vi "TEMOCR-Initialize Stimuli.vi"(0 "Data folder":path, 5 "Params":T2, 7 "AO in":T1, 11 "error in (no error)":errorcluster) -> (8 "AO out":T1, 15 "error out":errorcluster)   [LabVIEW 2015]
uses:
  Typedefs/TEMOCR-Parameters.ctl
  Typedefs/TEMOCR-Probe.ctl
  Typedefs/TEMOCR-Elicitor.ctl
  Human Studies/SFM Frontend/LV Source/Typedefs/HSTS-Transducer.ctl
  Typedefs/TEMOCR-Sequence.ctl
  Typedefs/TEMOCR-Analysis.ctl
  Typedefs/TEMOCR-AO Data.ctl
  Signal Synthesis VIs/3rd Generation/XControls/Stimulus Channel (G3)/Full Stimulus Channel Data.ctl
  Signal Synthesis VIs/3rd Generation/XControls/Waveform XControls/Waveform (G3)/Waveform Data.ctl
  Signal Synthesis VIs/3rd Generation/Waveform VIs/Waveform Enum (V3).ctl
  Signal Synthesis VIs/3rd Generation/XControls/Waveform XControls/Tone (G3)/Tone.Properties.ctl
  Signal Synthesis VIs/Waveform VIs/Pulse Train VIs/Pulse Train Params.ctl
  Signal Synthesis VIs/Waveform VIs/Pulse Train VIs/Pulse Polarity.ctl
  Signal Synthesis VIs/Waveform VIs/Pulse Train VIs/PT-Continuous State.ctl
  Signal Synthesis VIs/3rd Generation/Waveform VIs/Noise VIs/Noise (G3).ctl
  Signal Synthesis VIs/3rd Generation/Waveform VIs/Noise VIs/Noise (G3).Properties.ctl
  Signal Synthesis VIs/3rd Generation/Waveform VIs/Noise VIs/Noise (G3).Data.ctl
  Signal Synthesis VIs/Waveform VIs/File VIs/StimFile-Params.ctl
  Signal Synthesis VIs/Waveform VIs/FM Sweep VIs/FM Sweep Params.ctl
  Signal Synthesis VIs/Waveform VIs/Chirp Train VIs/Chirp Train.ctl
  Signal Synthesis VIs/Waveform VIs/Chirp Train VIs/Chirp Train Params.ctl
  Signal Synthesis VIs/Waveform VIs/Complex Tone VIs/CT-Params.ctl
  Signal Synthesis VIs/Waveform VIs/Complex Tone VIs/CT-Phase Enum.ctl
  Signal Synthesis VIs/Waveform VIs/Complex Tone VIs/CT-Runtime Data.ctl
  Signal Synthesis VIs/3rd Generation/XControls/Waveform XControls/FM Tone/Data.ctl
  Signal Synthesis VIs/3rd Generation/XControls/Waveform XControls/Vowel/Vowel.Properties.ctl
  Signal Synthesis VIs/3rd Generation/Waveform VIs/Ramp VIs/Ramp.Properties.ctl
  Signal Synthesis VIs/3rd Generation/XControls/Filter (G3)/Filter Data.ctl
  Signal Synthesis VIs/3rd Generation/XControls/Filter (G3)/Filter Type.ctl
  Signal Synthesis VIs/Filter VIs/Filter-Bandwidth Units.ctl
  Signal Synthesis VIs/Controls/Burst XCtl/Burst Data.ctl
  Signal Synthesis VIs/3rd Generation/XControls/Level (G3)/Level Data.ctl
  Signal Synthesis VIs/3rd Generation/XControls/Level (G3)/Level Units (G3).ctl
  Signal Synthesis VIs/3rd Generation/XControls/Advanced Options (G3)/Advanced Options (G3).ctl
  Signal Synthesis VIs/Modulation VIs/SAM VIs/SAM Params.ctl
  Signal Synthesis VIs/3rd Generation/Typedefs/Destination.ctl
  PXI DAQ VIs/DAQ Engine VIs/PXI Globals.vi
  Signal Synthesis VIs/Waveform VIs/Noise VIs/Noise-Globals.vi
  Utility VIs/Math VIs/LinSpace (start-stop-step).vi
  Utility VIs/Math VIs/dB to Linear (1D).vi
  Signal Synthesis VIs/3rd Generation/XControls/Waveform XControls/Tone (G3)/Tone (G3).xctl
  Signal Synthesis VIs/3rd Generation/XControls/Waveform XControls/FM Tone/FM Tone.xctl
  Signal Synthesis VIs/3rd Generation/XControls/Waveform XControls/Vowel/Vowel.xctl
  Signal Synthesis VIs/3rd Generation/XControls/Waveform XControls/Waveform (G3)/Waveform (G3).xctl
  Signal Synthesis VIs/3rd Generation/XControls/Filter (G3)/Filter (G3).xctl
  Signal Synthesis VIs/Controls/Burst XCtl/Burst Control.xctl
  Signal Synthesis VIs/3rd Generation/XControls/Level (G3)/Level (G3).xctl
  Signal Synthesis VIs/3rd Generation/XControls/Advanced Options (G3)/Advanced Options (G3).xctl
  Signal Synthesis VIs/3rd Generation/XControls/Stimulus Channel (G3)/Stimulus Channel (G3).xctl
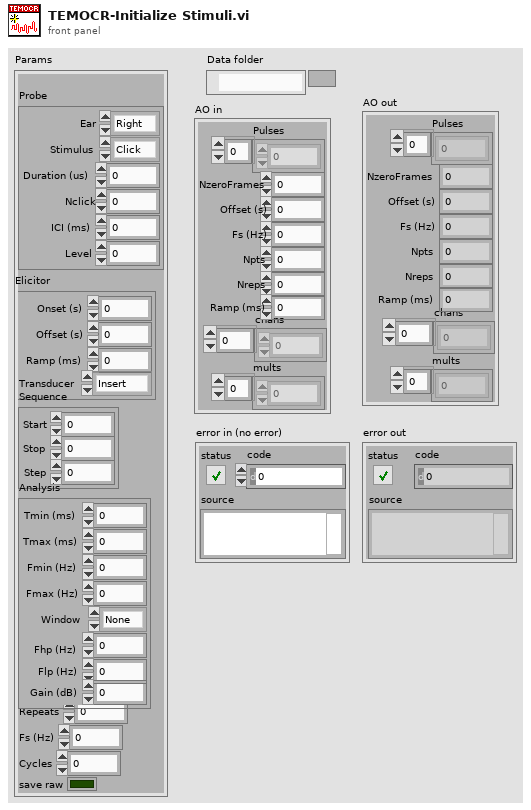
[diagram p1: front panel]
types:
  T1 = typedef "TEMOCR-AO Data.ctl" = cluster{"Pulses":dbl[], "Fs (Hz)":dbl, "Npts":i32, "mults":dbl[], "chans":i32[], "Nreps":i32, "NzeroFrames":i32, "Offset (s)":dbl, "Ramp (ms)":dbl}
  T2 = typedef "TEMOCR-Parameters.ctl" = cluster{"Probe":T3, "Elicitor":T4, "Sequence":T6, "Analysis":T7, "Repeats":i32, "Fs (Hz)":dbl, "Cycles":i32, "save raw":bool}
  T3 = typedef "TEMOCR-Probe.ctl" = cluster{"Ear":enum16{"Right", "Left"}, "Stimulus":enum16{"Click", "Chirp"}, "Duration (us)":dbl, "Nclick":i32, "ICI (ms)":dbl, "Level":dbl}
  T4 = typedef "TEMOCR-Elicitor.ctl" = cluster{"Onset (s)":dbl, "Offset (s)":dbl, "Ramp (ms)":dbl, "Transducer":T5}
  T5 = typedef "HSTS-Transducer.ctl" = enum16{"Insert", "TDH-39", "HD300", "ER-10X"}
  T6 = typedef "TEMOCR-Sequence.ctl" = cluster{"Start":dbl, "Stop":dbl, "Step":dbl}
  T7 = typedef "TEMOCR-Analysis.ctl" = cluster{"Tmin (ms)":dbl, "Tmax (ms)":dbl, "Fmin (Hz)":dbl, "Fmax (Hz)":dbl, "Window":enum16{"None", "Hanning", "Hamming"}, "Fhp (Hz)":dbl, "Flp (Hz)":dbl, "Gain (dB)":dbl}
  T8 = typedef "Filter (G3).xctl/Filter Type.ctl" = enum16{"OFF", "Lowpass", "Highpass", "Bandpass", "Bandstop"}
  T9 = typedef "Level (G3).xctl/Level Units (G3).ctl" = enum16{"dB atten", "dB SPL", "dB re 1 Vrms", "dB V/Hz½", "mW", "dB HL", "Volts", "dB mW"}
  T10 = typedef "Waveform Enum (V3).ctl" = enum16{"OFF", "Tone", "Noise", "Pulse Train", "File", "FM Sweep", "Chirp Train", "Complex Tone", "FM Tone", "Vowel", "Ramp"}
  T11 = typedef "Stimulus Channel (G3).xctl/Full Stimulus Channel Data.ctl" = cluster{"Waveform":T12, "Filter":T30, "Burst":T32, "Level":T33, "Name":string, "Advanced":T34, "SAM":T35, "Destination":T36}
  T12 = typedef "Waveform (G3).xctl/Waveform Data.ctl" = cluster{"Type":T10, "Tone":T13, "Pulse Train":T14, "Noise":T17, "File":T20, "FMSweep":T21, "Chirp Train":T22, "Complex Tone":cluster{"Params":T24, "Data":T26}, "FM":T27, "Vowel":T28, "Ramp":T29}
  T13 = typedef "Tone (G3).xctl/Tone.Properties.ctl" = cluster{"Frequency (kHz)":dbl, "Phase (cycles)":dbl, "Random phase":bool}
  T14 = typedef "Pulse Train Params.ctl" = cluster{"Pulse width (us)":dbl, "Pulse rate (Hz)":dbl, "Gap (ms)":dbl, "Polarity":T15, "PT State":T16, "Asynch":bool}
  T15 = typedef "Pulse Polarity.ctl" = enum16{"POS", "NEG", "POS-NEG", "NEG-POS"}
  T16 = typedef "PT-Continuous State.ctl" = cluster{"Template":dbl[], "Nperiod":i32, "Index":i32, "Pulse Rate (Hz)":dbl, "Phase (cycles)":dbl, "Noff":i32}
  T17 = typedef "Noise (G3).ctl" = cluster{"Properties":T18, "Data":T19}
  T18 = typedef "Noise (G3).Properties.ctl" = cluster{"InvFilt":bool, "Aweight":bool, "Seed":i32, "Tokens":i32, "Brickwall":bool}
  T19 = typedef "Noise (G3).Data.ctl" = cluster{"TokenNum":i32}
  T20 = typedef "StimFile-Params.ctl" = cluster{"Filename":path, "Signal":dbl[], "Channel":i32, "stream":bool, "offset":i32, "nreps":i32, "loops":i32}
  T21 = typedef "FM Sweep Params.ctl" = cluster{"Rate (oct/s)":dbl, "Fmin (Hz)":dbl, "Fmax (Hz)":dbl, "Ramp (ms)":dbl, "Linear":bool}
  T22 = typedef "Chirp Train.ctl" = cluster{"Params":T23, "Data":cluster{"WF":dbl[]}}
  T23 = typedef "Chirp Train Params.ctl" = cluster{"Fmin (kHz)":dbl, "Fmax (kHz)":dbl, "Compensate":bool, "Duration (ms)":dbl}
  T24 = typedef "CT-Params.ctl" = cluster{"F0 (Hz)":dbl, "Band":cluster{"Flow (Hz)":dbl, "Fhigh (Hz)":dbl}, "Phase":T25, "Min F0 (Hz)":dbl, "Max F0 (Hz)":dbl, "ContinRandPhase":bool, "Max peak factor":dbl, "Max mod depth":dbl, "MinHarmNum":i32, "MaxHarmNum":i32, "Level Mode":enum16{"per component", "overall rms"}, "% jitter":dbl}
  T25 = typedef "CT-Phase Enum.ctl" = enum16{"Cosine", "Random", "Alternating"}
  T26 = typedef "CT-Runtime Data.ctl" = cluster{"Ncomp":i32, "MinHarm":i32, "Phase":dbl[], "Amplitude":dbl[], "Npts/frame":i32, "Last F0":dbl, "Fmin":dbl, "Fmax":dbl, "Lslope":dbl, "randphase":bool, "overall rms":bool, "fmult":dbl[], "jittered":bool}
  T27 = typedef "FM Tone.xctl/Data.ctl" = cluster{"Carrier (kHz)":dbl, "ModRate (Hz)":dbl, "Depth (Hz)":dbl, "Phase (cycles)":dbl}
  T28 = typedef "Vowel.xctl/Vowel.Properties.ctl" = cluster{"Freqs":string, "Set level":enum16{"Total", "Per component"}, "Freq":dbl[], "weights":dbl[]}
  T29 = typedef "Ramp.Properties.ctl" = cluster{"Duration (ms)":dbl}
  T30 = typedef "Filter (G3).xctl/Filter Data.ctl" = cluster{"Type":T8, "CF (kHz)":dbl, "BW (kHz)":dbl, "Cascade":bool, "Quadrature":bool, "Scale Factor":dbl, "Stages":cluster{"IIR Filter":cluster{"filter structure":enum32{"IIR 2nd Order", "IIR 4th Order"}, "Reverse Coefficients":dbl[], "Forward Coefficients":dbl[]}, "State":dbl[]}[], "Class":enum16{"Elliptic", "Butterworth"}, "Order":i32, "BWUnits":T31}
  T31 = typedef "Filter-Bandwidth Units.ctl" = enum16{"Linear", "Octaves", "Min-Max"}
  T32 = typedef "Burst Control.xctl/Burst Data.ctl" = cluster{"Active":bool, "Delay (ms)":dbl, "Duration (ms)":dbl, "Ramp (ms)":dbl, "Rate (Hz)":dbl, "Trepeat (ms)":dbl, "Repeat":bool}
  T33 = typedef "Level (G3).xctl/Level Data.ctl" = cluster{"Level":dbl, "Units":T9, "Max":dbl, "Data":cluster{"Multiplier":dbl, "Cal File":path, "Cal":cluster{"Freq (Hz)":dbl[], "Mag (dB SPL)":dbl[], "Phase (deg)":dbl[]}, "audiogram":path}}
  T34 = typedef "Advanced Options (G3).xctl/Advanced Options (G3).ctl" = cluster{"AltPol":bool, "Var":string, "Expr":string}
  T35 = typedef "SAM Params.ctl" = cluster{"Active":bool, "Frequency (Hz)":dbl, "Depth":dbl, "Init Phase (cycles)":dbl, "phase (degrees)":dbl, "Asynch":bool}
  T36 = typedef "Destination.ctl" = cluster{"Name":string, "Num":i32}
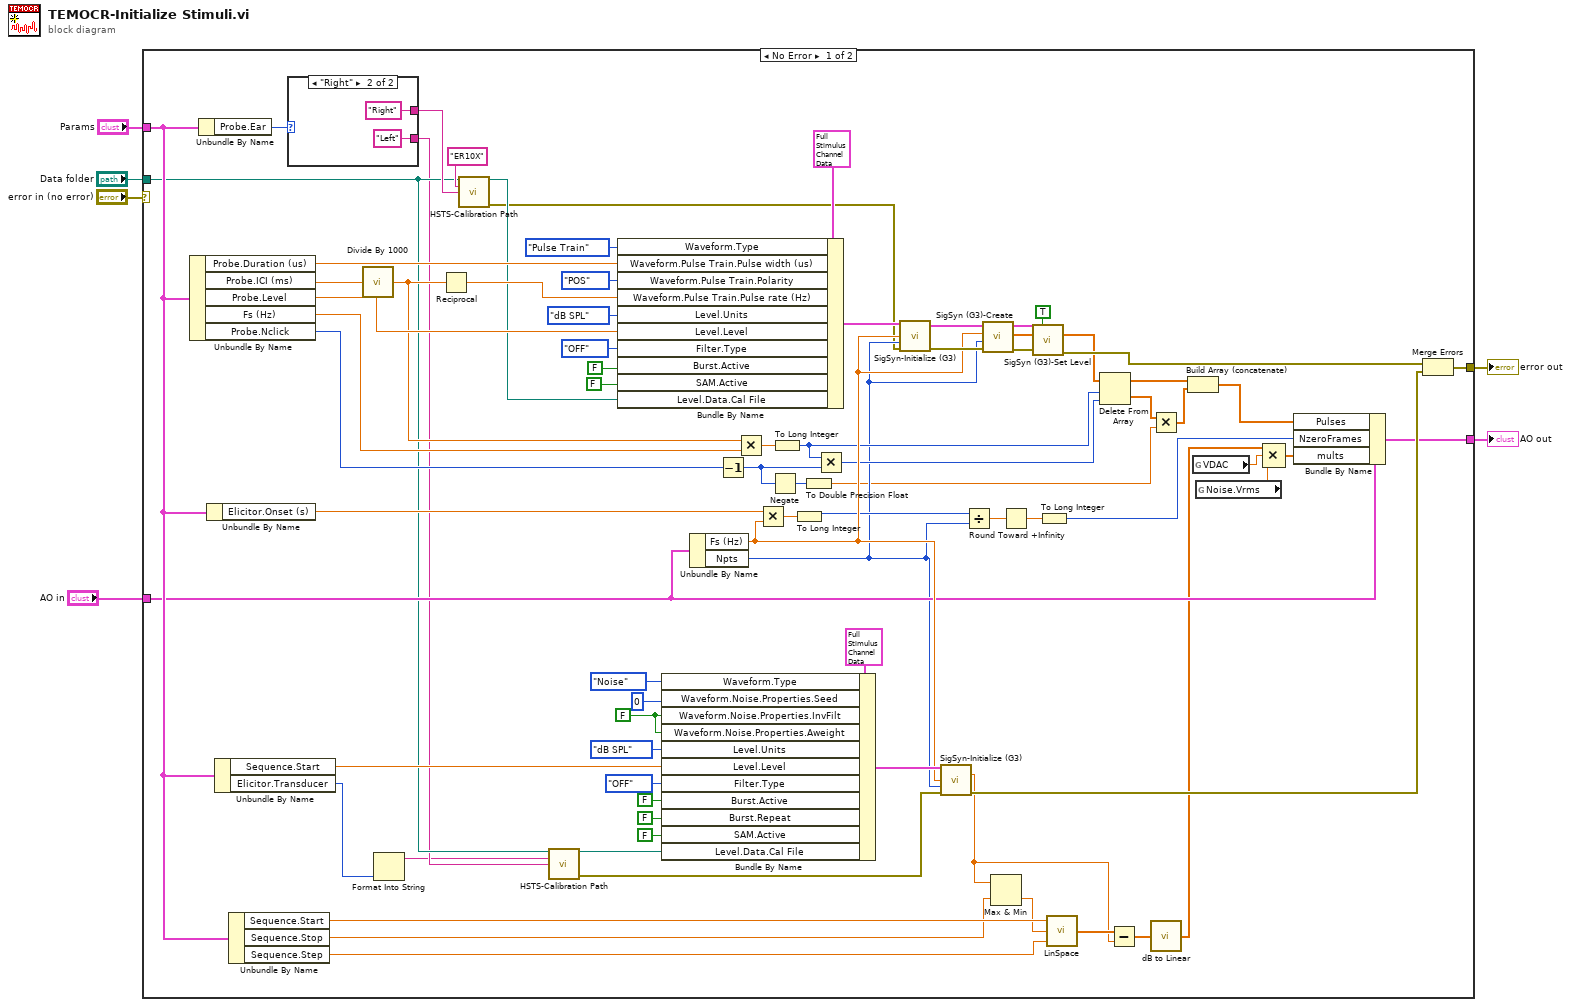
[diagram p0: block diagram]
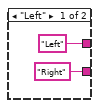
[diagram p2: hidden frame]
diagram:
  n1 = case shown="No Error" "error in (no error)" {
    selector: "error in (no error)" -> [_ w90]
    tunnel: "Data folder" -> [w11 _]
    tunnel: [w60 w90] -> w4
    tunnel: "Params" -> [w59 _]
    tunnel: [w51 _] -> w2
    tunnel: "AO in" -> [w49 _]
    frame No Error {
      w69 = FALSE ("Waveform.Noise.Properties.InvFilt")
      n2 = Unbundle By Name(w59) -> ("Probe.Duration (us)"=w39:dbl, "Probe.ICI (ms)"=w41:dbl, "Probe.Level"=w81:dbl, "Fs (Hz)"=w36:dbl, "Probe.Nclick"=w38:i32)
      n3 = Unbundle By Name(w59) -> ("Probe.Ear"=w17:enum16{"Right", "Left"})
      n4 = Unbundle By Name(w59) -> ("Elicitor.Onset (s)"=w27:dbl)
      n5 = Unbundle By Name(w59) -> ("Sequence.Start"=w67:dbl, "Elicitor.Transducer"=w7:T5)
      n6 = Unbundle By Name(w59) -> ("Sequence.Start"=w58:dbl, "Sequence.Stop"=w56:dbl, "Sequence.Step"=w57:dbl)
      n7 = case shown="\"Right\"" w17 {
        tunnel: ["Left" "Right"] -> w16
        tunnel: ["Right" "Left"] -> w9
        frame "Left" {
        }
        frame "Right" {
        }
      }
      n8 = call "Divide By 1000.vi"("X"=w41) -> ("X/1000"=w37:dbl)
      n9 = Format Into String(w7) -> (resulting string=w8:string)  [unwired: 3 in, 1 out]
      n10 = Reciprocal(x=w37) -> (1/x=w40:dbl)
      n11 = call "HSTS-Calibration Path.vi"("Data Folder"=w11, "Speaker"="ER10X", "Side"=w16) -> ("Cal Path"=w14:path, "error out"=w13:errorcluster)  [unwired: 11 in]
      n12 = call "HSTS-Calibration Path.vi"("Data Folder"=w11, "Speaker"=w8, "Side"=w9) -> ("Cal Path"=w12:path, "error out"=w10:errorcluster)  [unwired: 11 in]
      n13 = Bundle By Name(cluster=T11 {"Waveform"={"Type"=enum."Tone", "Tone"={"Frequency (kHz)"=0.0, "Phase (cycles)"=0.0, "Random phase"=FALSE}, "Pulse Train"={"Pulse width (us)"=0.0, "Pulse rate (Hz)"=0.0, "Gap (ms)"=0.0, "Polarity"=enum."POS", "PT State"={"Template"=[], "Nperiod"=0, "Index"=0, "Pulse Rate (Hz)"=0.0, "Phase (cycles)"=0.0, "Noff"=0}, "Asynch"=FALSE}, "Noise"={"Properties"={"InvFilt"=FALSE, "Aweight"=FALSE, "Seed"=0, "Tokens"=0, "Brickwall"=FALSE}, "Data"={"TokenNum"=0}}, "File"={"Filename"=path "", "Signal"=[], "Channel"=0, "stream"=FALSE, "offset"=0, "nreps"=0, "loops"=0}, "FMSweep"={"Rate (oct/s)"=0.0, "Fmin (Hz)"=0.0, "Fmax (Hz)"=0.0, "Ramp (ms)"=0.0, "Linear"=FALSE}, "Chirp Train"={"Params"={"Fmin (kHz)"=4.0, "Fmax (kHz)"=64.0, "Compensate"=FALSE, "Duration (ms)"=2.0}, "Data"={"WF"=[]}}, "Complex Tone"={"Params"={"F0 (Hz)"=0.0, "Band"={"Flow (Hz)"=0.0, "Fhigh (Hz)"=0.0}, "Phase"=enum."Cosine", "Min F0 (Hz)"=0.0, "Max F0 (Hz)"=0.0, "ContinRandPhase"=FALSE, "Max peak factor"=inf, "Max mod depth"=2.0, "MinHarmNum"=0, "MaxHarmNum"=0, "Level Mode"=enum."per component", "% jitter"=0.0}, "Data"={"Ncomp"=0, "MinHarm"=0, "Phase"=[], "Amplitude"=[], "Npts/frame"=0, "Last F0"=0.0, "Fmin"=0.0, "Fmax"=0.0, "Lslope"=0.0, "randphase"=FALSE, "overall rms"=FALSE, "fmult"=[], "jittered"=FALSE}}, "FM"={"Carrier (kHz)"=0.0, "ModRate (Hz)"=0.0, "Depth (Hz)"=0.0, "Phase (cycles)"=0.0}, "Vowel"={"Freqs"="", "Set level"=enum."Total", "Freq"=[], "weights"=[]}, "Ramp"={"Duration (ms)"=0.0}}, "Filter"={"Type"=enum."Lowpass", "CF (kHz)"=0.0, "BW (kHz)"=0.0, "Cascade"=FALSE, "Quadrature"=FALSE, "Scale Factor"=0.0, "Stages"=[], "Class"=enum."Elliptic", "Order"=0, "BWUnits"=enum."Linear"}, "Burst"={"Active"=FALSE, "Delay (ms)"=0.0, "Duration (ms)"=0.0, "Ramp (ms)"=0.0, "Rate (Hz)"=0.0, "Trepeat (ms)"=0.0, "Repeat"=FALSE}, "Level"={"Level"=0.0, "Units"=enum."dB atten", "Max"=0.0, "Data"={"Multiplier"=0.0, "Cal File"=path "", "Cal"={"Freq (Hz)"=[], "Mag (dB SPL)"=[], "Phase (deg)"=[]}, "audiogram"=path ""}}, "Name"="", "Advanced"={"AltPol"=FALSE, "Var"="", "Expr"=""}, "SAM"={"Active"=FALSE, "Frequency (Hz)"=0.0, "Depth"=0.0, "Init Phase (cycles)"=0.0, "phase (degrees)"=0.0, "Asynch"=FALSE}, "Destination"={"Name"="", "Num"=0}} ("Stimulus"), "Waveform.Type"=Waveform_Enum_(V3)."Pulse Train", "Waveform.Pulse Train.Pulse width (us)"=w39, "Waveform.Pulse Train.Polarity"=Pulse_Polarity."POS", "Waveform.Pulse Train.Pulse rate (Hz)"=w40, "Level.Units"=Level_Units_(G3)."dB SPL", "Level.Level"=w81, "Filter.Type"=Filter_Type."OFF", "Burst.Active"=FALSE, "SAM.Active"=FALSE, "Level.Data.Cal File"=w14) -> (w77:T11)
      n14 = Bundle By Name(cluster=T11 {"Waveform"={"Type"=enum."Tone", "Tone"={"Frequency (kHz)"=0.0, "Phase (cycles)"=0.0, "Random phase"=FALSE}, "Pulse Train"={"Pulse width (us)"=0.0, "Pulse rate (Hz)"=0.0, "Gap (ms)"=0.0, "Polarity"=enum."POS", "PT State"={"Template"=[], "Nperiod"=0, "Index"=0, "Pulse Rate (Hz)"=0.0, "Phase (cycles)"=0.0, "Noff"=0}, "Asynch"=FALSE}, "Noise"={"Properties"={"InvFilt"=FALSE, "Aweight"=FALSE, "Seed"=0, "Tokens"=0, "Brickwall"=FALSE}, "Data"={"TokenNum"=0}}, "File"={"Filename"=path "", "Signal"=[], "Channel"=0, "stream"=FALSE, "offset"=0, "nreps"=0, "loops"=0}, "FMSweep"={"Rate (oct/s)"=0.0, "Fmin (Hz)"=0.0, "Fmax (Hz)"=0.0, "Ramp (ms)"=0.0, "Linear"=FALSE}, "Chirp Train"={"Params"={"Fmin (kHz)"=4.0, "Fmax (kHz)"=64.0, "Compensate"=FALSE, "Duration (ms)"=2.0}, "Data"={"WF"=[]}}, "Complex Tone"={"Params"={"F0 (Hz)"=0.0, "Band"={"Flow (Hz)"=0.0, "Fhigh (Hz)"=0.0}, "Phase"=enum."Cosine", "Min F0 (Hz)"=0.0, "Max F0 (Hz)"=0.0, "ContinRandPhase"=FALSE, "Max peak factor"=inf, "Max mod depth"=2.0, "MinHarmNum"=0, "MaxHarmNum"=0, "Level Mode"=enum."per component", "% jitter"=0.0}, "Data"={"Ncomp"=0, "MinHarm"=0, "Phase"=[], "Amplitude"=[], "Npts/frame"=0, "Last F0"=0.0, "Fmin"=0.0, "Fmax"=0.0, "Lslope"=0.0, "randphase"=FALSE, "overall rms"=FALSE, "fmult"=[], "jittered"=FALSE}}, "FM"={"Carrier (kHz)"=0.0, "ModRate (Hz)"=0.0, "Depth (Hz)"=0.0, "Phase (cycles)"=0.0}, "Vowel"={"Freqs"="", "Set level"=enum."Total", "Freq"=[], "weights"=[]}, "Ramp"={"Duration (ms)"=0.0}}, "Filter"={"Type"=enum."Lowpass", "CF (kHz)"=0.0, "BW (kHz)"=0.0, "Cascade"=FALSE, "Quadrature"=FALSE, "Scale Factor"=0.0, "Stages"=[], "Class"=enum."Elliptic", "Order"=0, "BWUnits"=enum."Linear"}, "Burst"={"Active"=FALSE, "Delay (ms)"=0.0, "Duration (ms)"=0.0, "Ramp (ms)"=0.0, "Rate (Hz)"=0.0, "Trepeat (ms)"=0.0, "Repeat"=FALSE}, "Level"={"Level"=0.0, "Units"=enum."dB atten", "Max"=0.0, "Data"={"Multiplier"=0.0, "Cal File"=path "", "Cal"={"Freq (Hz)"=[], "Mag (dB SPL)"=[], "Phase (deg)"=[]}, "audiogram"=path ""}}, "Name"="", "Advanced"={"AltPol"=FALSE, "Var"="", "Expr"=""}, "SAM"={"Active"=FALSE, "Frequency (Hz)"=0.0, "Depth"=0.0, "Init Phase (cycles)"=0.0, "phase (degrees)"=0.0, "Asynch"=FALSE}, "Destination"={"Name"="", "Num"=0}} ("Stimulus"), "Waveform.Type"=Waveform_Enum_(V3)."Noise", "Waveform.Noise.Properties.Seed"=0, "Waveform.Noise.Properties.InvFilt"=w69, "Waveform.Noise.Properties.Aweight"=w69, "Level.Units"=Level_Units_(G3)."dB SPL", "Level.Level"=w67, "Filter.Type"=Filter_Type."OFF", "Burst.Active"=FALSE, "Burst.Repeat"=FALSE, "SAM.Active"=FALSE, "Level.Data.Cal File"=w12) -> (w62:T11)
      n15 = Unbundle By Name(w49) -> ("Fs (Hz)"=w50:dbl, "Npts"=w25:i32)
      n16 = Decrement(x=w38) -> (x-1=w20:i32)
      n17 = Multiply(x=w37, y=w36) -> (x*y=w73:dbl)
      n18 = Multiply(x=w27, y=w50) -> (x*y=w74:dbl)
      n19 = Negate(x=w20) -> (-x=w31:i32)
      n20 = To Long Integer(number=w73) -> (32bit integer=w33:i32)
      n21 = To Long Integer(number=w74) -> (32bit integer=w26:i32)
      n22 = To Double Precision Float(number=w31) -> (double precision float=w18:dbl)
      n23 = Multiply(x=w33, y=w20) -> (x*y=w34:i32)
      n24 = call "SigSyn-Initialize (G3).vi"("Stimulus Channel"=w77, "Sampling rate (Hz)"=w50, "Npts"=w25, "error in (no error)"=w13) -> ("Stimulus Channel out"=w75:T11, "error out"=w76:errorcluster)  [unwired: 9 in, 1 out]
      n25 = call "SigSyn-Initialize (G3).vi"("Stimulus Channel"=w62, "Sampling rate (Hz)"=w50, "Npts"=w25, "error in (no error)"=w10) -> ("Max Level"=w53:dbl, "error out"=w61:errorcluster)  [unwired: 9 in, 1 out]
      n26 = Divide(x=w26, y=w25) -> (x/y=w24:dbl)
      n27 = call "SigSyn (G3)-Create.vi"("error in (no error)"=w76, "Npts"=w25, "Sampling Rate (Hz)"=w50, "Stimulus Channel"=w75) -> ("error out"=w43:errorcluster, "Waveform"=w44:dbl[], "Stimulus Channel out"=w45:T11)  [unwired: 4 in, 1 out]
      n28 = Max & Min(x=w53, y=w56) -> (min(x,y)=w55:dbl)  [unwired: 1 out]
      n29 = Round Toward +Infinity(x=w24) -> (ceil(x): smallest int >= x=w23:dbl)
      n30 = call "SigSyn (G3)-Set Level.vi"("StimChans In"=w45, "Apply multiplier? (F)"=TRUE, "Waveform in"=w44, "error in (no error)"=w43) -> ("Waveform out"=w35:dbl[], "error out"=w42:errorcluster)  [unwired: 7 in, 3 out]
      n31 = To Long Integer(number=w23) -> (32bit integer=w22:i32)
      n32 = call-poly "LinSpace.vi"("Step"=w57, "Stop"=w55, "Start"=w58) -> ("Array"=w54:dbl[])  [unwired: 1 in, 1 out]
      n33 = Delete From Array(array=w35, length=w33, index=w34) -> (deleted portion=w32:dbl[], array with subset deleted=w30:dbl[])
      n34 = Subtract(x=w54, y=w53) -> (x-y=w52:dbl[])
      n35 = Multiply(x=w32, y=w18) -> (x*y=w29:dbl[])
      n36 = call-poly "dB to Linear.vi"("dB"=w52) -> ("linear"=w48:dbl[])
      n37 = Build Array (concatenate)(w30, w29) -> (w28:dbl[])
      n38 = global read "PXI Globals.vi" "VDAC"() -> (w46:dbl)
      n39 = global read "Noise-Globals.vi" "Noise.Vrms"() -> (w21:dbl)
      n40 = Compound Arithmetic op=MULTIPLY(w48, w46, w21) -> (w47:dbl[])
      n41 = Bundle By Name(cluster=w49, "Pulses"=w28, "NzeroFrames"=w22, "mults"=w47) -> (w51:T1)
      n42 = Merge Errors(w42, w61) -> (w60:errorcluster)
    }
    frame Error {
    }
  }
  "error out" <- w4
  "AO out" <- w2
